vi "TCP Read select.vi"(7 "mode (standard)":T1(ring), 8 "error in (no error)":errorcluster, 9 "timeout":i32, 10 "bytes to read":i32, 11 "connection ID":refnum<k5>) -> (0 "error out":errorcluster, 1 "timed out?":bool, 2 "data":string)   [LabVIEW 2021, in "TCP Shared Components.lvlib"]
doc: "This function reads a TCP packet from the bus and checks for errors. It is a wrapper for standard functionality."
uses:
  TCP Shared Components.lvlib
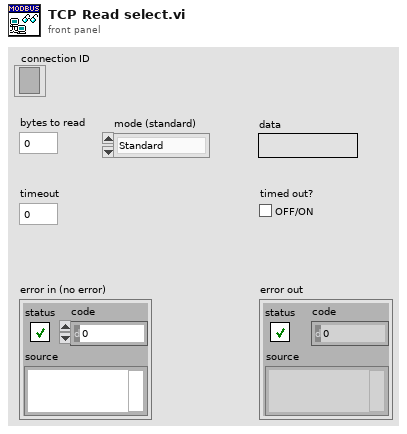
[diagram p1: front panel]
types:
  T1 = enum16{"Standard", "Buffered", "CRLF", "Immediate"}
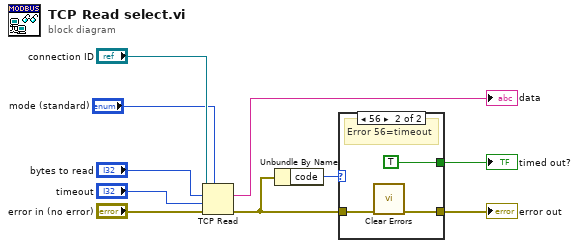
[diagram p0: block diagram]
diagram:
  n1 = TCP Read(connection ID="connection ID", bytes to read="bytes to read", error in (no error)="error in (no error)", 7:"mode (standard)", 9:"timeout") -> (data out=→"data":string, error out=w2:errorcluster)  [unwired: 1 out]
  n2 = Unbundle By Name(w2) -> ("code"=w1:i32)
  n3 = case shown="56" w1 {
    tunnel: w2 -> [w11 w13]
    tunnel: [w11 w12] -> w10
    tunnel: [_ TRUE] -> w5
    frame 0, Default {
    }
    frame 56 {
      # "Error 56=timeout"
      n4 = call <vilib>:"Clear Errors.vi"("error in (no error)"=w13) -> ("error out"=w12:errorcluster)  [unwired: 5 in, 1 out]
    }
  }
  "error out" <- w10
  "timed out?" <- w5
